vi "FPGA_target_set_stop_output.vi"(9 "connector0_data":T1, 11 "connector1_data":T1) -> ()   [LabVIEW 2014]
doc: "writes the pattern data to the outputs in case the pattern output is stopped"
uses:
  FPGA_32BitPattern_data_type.ctl
  <vilib>/rvi/eio/common/nirviEmuTemplateMethod_errors.vi
  <vilib>/eio/EIONode/EIONode.xnode
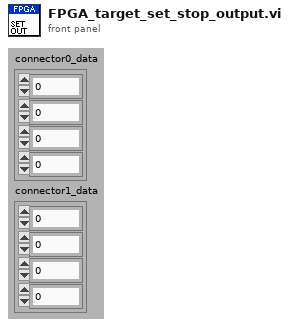
[diagram p1: front panel]
types:
  T1 = typedef "FPGA_32BitPattern_data_type.ctl" = cluster{"port0":u8, "port1":u8, "port2":u8, "port3":u8}
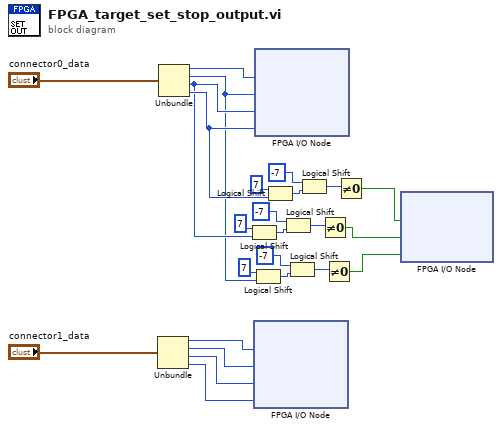
[diagram p0: block diagram]
diagram:
  n1 = Unbundle("connector1_data") -> ("port0"=w19:u8, "port1"=w20:u8, "port2"=w21:u8, "port3"=w22:u8)
  n2 = Unbundle("connector0_data") -> ("port0"=w23:u8, "port1"=w1:u8, "port2"=w2:u8, "port3"=w3:u8)
  n3 = Logical Shift(y=i16 7, x=w2) -> (x << y=w12:u8)
  n4 = Logical Shift(y=i16 7, x=w1) -> (x << y=w7:u8)
  n5 = xnode ("FPGA I/O Node")("DO_56-63"=w19, "DO_48-55"=w20, "DO_40-47"=w21, "DO_32-39"=w22) -> ()  [unwired: 4 in, 4 out]
  n6 = xnode ("FPGA I/O Node")("DO_24-31"=w23, "DO_16-23"=w1, "DO_08-15"=w2, "DO_00-07"=w3) -> ()  [unwired: 4 in, 4 out]
  n7 = Logical Shift(y=i16 7, x=w3) -> (x << y=w17:u8)
  n8 = Logical Shift(y=i16 -7, x=w12) -> (x << y=w10:u8)
  n9 = Logical Shift(y=i16 -7, x=w7) -> (x << y=w5:u8)
  n10 = Logical Shift(y=i16 -7, x=w17) -> (x << y=w15:u8)
  n11 = Not Equal To 0?(x=w10) -> (x != 0?=w9:bool)
  n12 = Not Equal To 0?(x=w5) -> (x != 0?=w4:bool)
  n13 = Not Equal To 0?(x=w15) -> (x != 0?=w14:bool)
  n14 = xnode "FPGA I/O Node"("PXI_Trig0"=w14, "PXI_Trig1"=w9, "PXI_Trig2"=w4) -> ()  [unwired: 3 in, 3 out]
